vi "Verify Minor Frame SubRoutine.vi"(5 "Instruction ID":i32, 6 "Pointers":T1={"Major Command Pointer"=2206, "Major Data Pointer"=2206, "Minor Command Pointer"=2206, "Minor Data Pointer"=2206}, 7 "Target IC (1-8)":u8, 8 "error in (no error)":errorcluster, 11 "BC Major Frame in":refnum<class "BC Major Frame.lvclass">) -> (0 "error out":errorcluster, 3 "BC Major Frame out":refnum<class "BC Major Frame.lvclass">, 4 "Pointers out":T1={"Major Command Pointer"=0, "Major Data Pointer"=0, "Minor Command Pointer"=2206, "Minor Data Pointer"=2206})   [LabVIEW 2016, in "BC Major Frame.lvclass"]
uses:
  BC Major Frame.lvclass
  Data Pointers.ctl
  Frames & Messages/TypeDefs/BC Op Codes - Verbose.ctl
  Frames & Messages/TypeDefs/BC Condition Codes.ctl
  BC Major Frame.lvclass/BC Major Frame.ctl
  Dependencies/Registry/Registry.lvclass/Registry.ctl
  PPLs/FPGA Interface.lvlibp/FPGA Interface/FPGA Interface.lvclass
  BCI-1553 API.lvlib
  Dependencies/Registry/Registry.lvclass
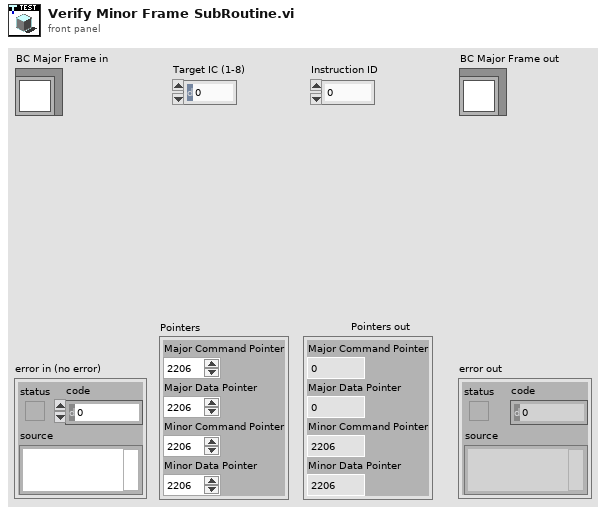
[diagram p1: front panel]
types:
  T1 = typedef "Data Pointers.ctl" = cluster{"Major Command Pointer":u16, "Major Data Pointer":u16, "Minor Command Pointer":u16, "Minor Data Pointer":u16}
  T2 = typedef "BCI-1553 API.lvlib/BC Condition Codes.ctl" = enum16{"GP0 == 1 || LT", "GP1 == 1 || NE", "GP2 == 1", "GP3 == 1", "GP4 == 1", "GP5 == 1", "GP6 == 1", "GP7 == 1", "NORESP", "FMTERR", "GOODBLOCK", "MSKSTATSET", "BADMSG", "1RETRY", "2RETRY", "ALWAYS"}
  T3 = typedef "BCI-1553 API.lvlib/BC Op Codes - Verbose.ctl" = enum16{"EXECUTE MSG", "EXECUTE MSG GO", "JUMP", "CALL SUBROUTINE", "RETURN", "INTERRUPT REQUEST", "HALT", "DELAY", "WAIT FRAME TIMER = 0", "COMPARE FRAME TIMER", "COMPARE MSG TIMER", "LOAD TIME TAG CTR", "LOAD TIME TAG CTR HI", "LOAD FRAME TIMER", "START FRAME TIMER", "PUSH TIME TAG COUNT", "PUSH TIME TAG COUNT HI", "PUSH TIME TAG COUNT BOTH", "PUSH BLOCK STATUS WORD", "PUSH CURRENT VALUE", "PUSH INDIRECT", "WAIT EXT TRIGGER", "EXECUTE AND FLIP", "EXECUTE, FLIP, GO", "WRITE VALUE TO WMI", "WRITE VALUE TO MEM", "DECREMENT RAM, SKIP", "FLAG"}
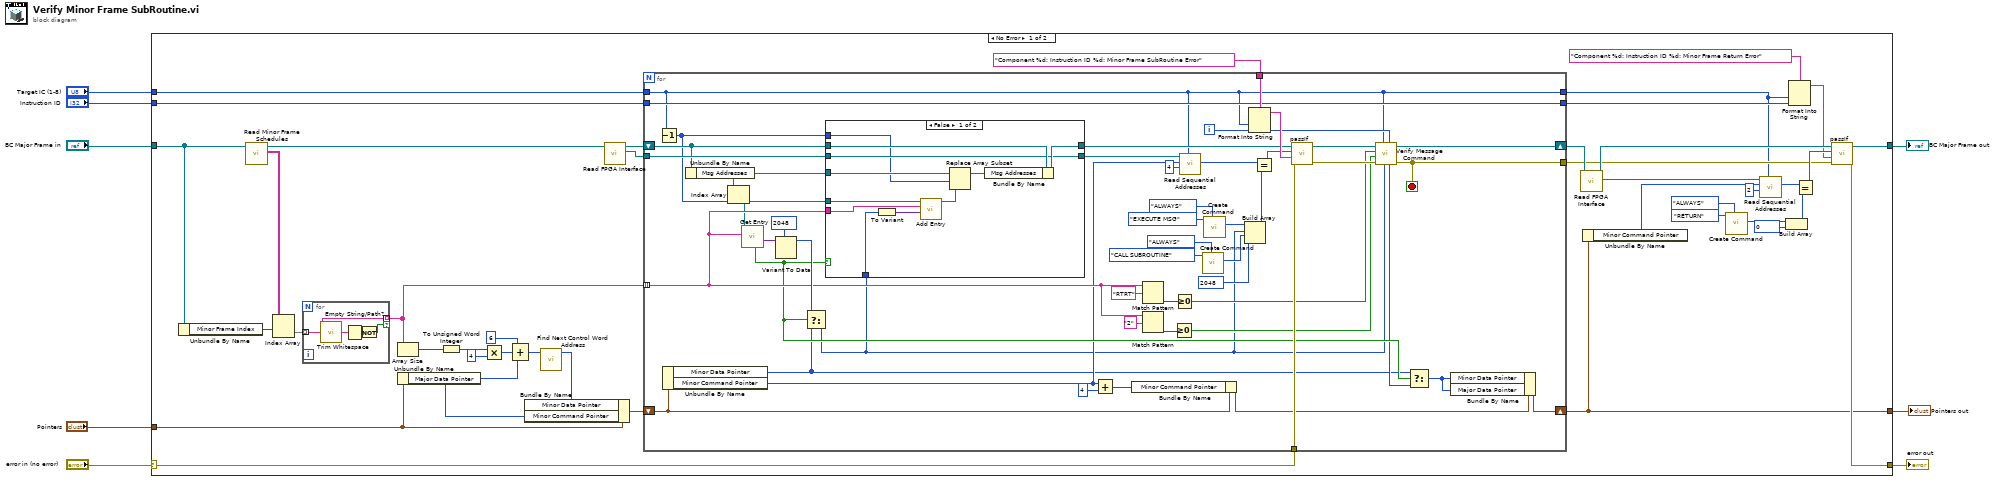
[diagram p0: block diagram]
diagram:
  n1 = case shown="No Error" "error in (no error)" {
    selector: "error in (no error)" -> [w47 w118]
    tunnel: [w30 w118] -> w7
    tunnel: [w29 w117] -> w5
    tunnel: "BC Major Frame in" -> [w50 w117]
    tunnel: "Target IC (1-8)" -> [w45 _]
    tunnel: "Instruction ID" -> [w44 _]
    tunnel: "Pointers" -> [w12 _]
    tunnel: [w10 _] -> w1
    frame No Error {
      n2 = Unbundle By Name(w50) -> ("Minor Frame Index"=w48:i32)
      n3 = call-dynamic "Read Minor Frame Schedules.vi"("1553 Test in"=w50) -> ("Minor Frame Schedules"=w49:string[][], "1553 Test out"=w35:refnum<class "BC Major Frame.lvclass">)  [unwired: 8 in, 1 out]
      n4 = Index Array(array=w49, index (row)=w48) -> (element=w38:string[])  [unwired: 1 in]
      n5 = for {
        tunnel: w38 -> [w115] mode=indexing
        tunnel: [w115] -> w37 mode=indexing if=w113
        n6 = call <vilib>:"Trim Whitespace.vi"("string"=w115) -> ("trimmed string"=w116:string)  [unwired: 1 in]
        n7 = Empty String/Path?(string/path=w116) -> (empty?=w114:bool)
        n8 = Not(x=w114) -> (.not. x?=w113:bool)
      }
      n9 = Array Size(array=w37) -> (size(s)=w36:i32)
      n10 = Unbundle By Name(w12) -> ("Major Data Pointer"=w11:u16)
      n11 = To Unsigned Word Integer(number=w36) -> (unsigned 16bit integer=w39:u16)
      n12 = Multiply(x=w39, y=u16 4) -> (x*y=w41:u16)
      n13 = Compound Arithmetic op=ADD(u16 6 ("value"), w41, w11) -> (w43:u16)
      n14 = call "Find Next Control Word Address.vi"("Starting Address"=w43) -> ("0xHHHX Address"=w14:u16)  [unwired: 10 in]
      n15 = Bundle By Name(cluster=w12, "Minor Data Pointer"=w14, "Minor Command Pointer"=w11) -> (w13:T1)
      n16 = call-dynamic "Read FPGA Interface.vi"("1553 Test in"=w35) -> ("FPGA Interface"=w33:refnum<class "FPGA Interface.lvclass">, "1553 Test out"=w34:refnum<class "BC Major Frame.lvclass">)  [unwired: 8 in, 1 out]
      n17 = for {
        shift-right: [w99] -> w24
        shift-left: w34 -> [w65]
        tunnel: [w98] -> w19
        tunnel: w47 -> [w94]
        tunnel: w37 -> [w69] mode=indexing
        tunnel: "Component %d: Instruction ID %d: Minor Frame SubRoutine Error" ("message (\"\")") -> [w92]
        tunnel: w45 -> [w62]
        tunnel: w44 -> [w74]
        tunnel: w33 -> [w67]
        tunnel: [w62] -> w15
        tunnel: [w74] -> w17
        shift-right: [w57] -> w10
        shift-left: w13 -> [w54]
        i -> [w73]
        stop <- w98 stop-if-true
        n18 = Decrement(x=w62) -> (x-1=w59:u8)
        n19 = Unbundle By Name(w54) -> ("Minor Data Pointer"=w56:u16, "Minor Command Pointer"=w58:u16)
        n20 = Unbundle By Name(w65) -> ("Msg Addresses"=w60:refnum<class "Registry.lvclass">[])
        n21 = Index Array(array=w60, index=w59) -> (element=w61:refnum<class "Registry.lvclass">)
        n22 = call "Get Entry.vi"("Key"=w69, "Registry in"=w61) -> ("Value"=w72:variant, "Found?"=w64:bool)  [unwired: 6 in, 2 out]
        n23 = Variant To Data(type=u16 2048, Variant=w72) -> (data=w70:u16)  [unwired: 1 in, 1 out]
        n24 = Select(t=w70, s=w64, f=w56) -> (s? t:f=w52:u16)
        n25 = case shown="False" w64 {
          tunnel: w69 -> [w110 _]
          tunnel: w52 -> [w109 _]
          tunnel: [w105 w112] -> w68
          tunnel: w67 -> [w105 w112]
          tunnel: [w106 w111] -> w66
          tunnel: w65 -> [w107 w111]
          tunnel: w59 -> [w100 _]
          tunnel: w61 -> [w104 _]
          tunnel: w60 -> [w103 _]
          frame False {
            n26 = To Variant(anything=w109) -> (Variant=w108:variant)
            n27 = call "Add Entry.vi"("Value"=w108, "Key"=w110, "Registry in"=w104) -> ("Registry out"=w101:refnum<class "Registry.lvclass">)  [unwired: 6 in, 2 out]
            n28 = Replace Array Subset(array=w103, new element=w101, index=w100) -> (w102:refnum<class "Registry.lvclass">[])
            n29 = Bundle By Name(cluster=w107, "Msg Addresses"=w102) -> (w106:refnum<class "BC Major Frame.lvclass">)
          }
          frame True {
          }
        }
        n30 = Add(x=w58, y=u16 4) -> (x+y=w55:u16)
        n31 = Bundle By Name(cluster=w54, "Minor Command Pointer"=w55) -> (w53:T1)
        n32 = Match Pattern(string=w69, regular expression="RTRT") -> (offset past match=w80:i32)  [unwired: 1 in, 3 out]
        n33 = Match Pattern(string=w69, regular expression="2") -> (offset past match=w77:i32)  [unwired: 1 in, 3 out]
        n34 = Greater Or Equal To 0?(x=w77) -> (x >= 0?=w75:bool)
        n35 = Greater Or Equal To 0?(x=w80) -> (x >= 0?=w76:bool)
        n36 = call-dynamic "Read Sequential Addresses.vi"("Target IC (1-8)"=w62, "Addresses to Read"=u16 4, "Starting Address"=w58, "FPGA Interface in"=w68) -> ("Data"=w82:u16[])  [unwired: 6 in, 1 out]
        n37 = call "Create Command.vi"("Condition"=BC_Condition_Codes."ALWAYS", "Op Code"=BC_Op_Codes_-_Verbose."CALL SUBROUTINE") -> ("Instruction"=w86:u16)  [unwired: 8 in, 1 out]
        n38 = call "Create Command.vi"("Condition"=BC_Condition_Codes."ALWAYS", "Op Code"=BC_Op_Codes_-_Verbose."EXECUTE MSG") -> ("Instruction"=w85:u16)  [unwired: 8 in, 1 out]
        n39 = Build Array(w85, w52, w86, u16 2048) -> (w83:u16[])
        n40 = Format Into String(format string=w92, w62, w73) -> (resulting string=w91:string)  [unwired: 2 in, 1 out]
        n41 = Equal?(x=w82, y=w83) -> (x = y?=w81:bool)
        n42 = call-dynamic "passIf.vi"("error in (no error)"=w94, "message (\"\")"=w91, "pass"=w81, "TestCase in"=w66) -> ("error out"=w93:errorcluster, "TestCase out"=w95:refnum<class "BC Major Frame.lvclass">)  [unwired: 6 in]
        n43 = call-dynamic "Verify Message Command.vi"("Instruction ID"=w73, "Cmd Address"=w52, "Target IC (1-8)"=w62, "error in (no error)"=w93, "Transmit?"=w75, "RT-RT?"=w76, "BC Major Frame in"=w95) -> ("error out"=w98:errorcluster, "BC Major Frame out"=w99:refnum<class "BC Major Frame.lvclass">, "Post-Data Address"=w63:u16)  [unwired: 2 in]
        n44 = Select(t=w56, s=w64, f=w63) -> (s? t:f=w51:u16)
        n45 = Bundle By Name(cluster=w53, "Minor Data Pointer"=w51, "Major Data Pointer"=w51) -> (w57:T1)
      }
      n46 = call-dynamic "Read FPGA Interface.vi"("1553 Test in"=w24) -> ("FPGA Interface"=w31:refnum<class "FPGA Interface.lvclass">, "1553 Test out"=w23:refnum<class "BC Major Frame.lvclass">)  [unwired: 8 in, 1 out]
      n47 = Unbundle By Name(w10) -> ("Minor Command Pointer"=w9:u16)
      n48 = call "Create Command.vi"("Condition"=BC_Condition_Codes."ALWAYS", "Op Code"=BC_Op_Codes_-_Verbose."RETURN") -> ("Instruction"=w26:u16)  [unwired: 8 in, 1 out]
      n49 = call-dynamic "Read Sequential Addresses.vi"("Target IC (1-8)"=w15, "Addresses to Read"=u16 2, "Starting Address"=w9, "FPGA Interface in"=w31) -> ("Data"=w32:u16[])  [unwired: 6 in, 1 out]
      n50 = Build Array(w26, u16 0 ("element")) -> (w21:u16[])
      n51 = Format Into String(format string="Component %d: Instruction ID %d: Minor Frame Return Error" ("message (\"\")"), w15, w17) -> (resulting string=w16:string)  [unwired: 2 in, 1 out]
      n52 = Equal?(x=w32, y=w21) -> (x = y?=w20:bool)
      n53 = call-dynamic "passIf.vi"("error in (no error)"=w19, "message (\"\")"=w16, "pass"=w20, "TestCase in"=w23) -> ("error out"=w30:errorcluster, "TestCase out"=w29:refnum<class "BC Major Frame.lvclass">)  [unwired: 6 in]
    }
    frame Error {
    }
  }
  "error out" <- w7
  "BC Major Frame out" <- w5
  "Pointers out" <- w1
